vi "PXI Multipliers to AO Gains.vi"   [LabVIEW 2020]
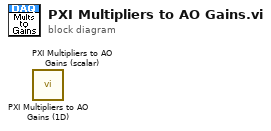
[diagram p0: block diagram]
diagram:
  n1 = call "PXI Multipliers to AO Gains (1D).vi"() -> ()  [unwired: 13 in, 3 out]
  n2 = call "PXI Multipliers to AO Gains (scalar).vi"() -> ()  [unwired: 13 in, 3 out]
